vi "Method_Const.vi"(4 "Value":cxt, 5 "Input A":T1) -> (1 "Result":T1)   [LabVIEW 2021, in "Multiply_CPLX_EXT.lvclass"]
uses:
  Multiply_CPLX_EXT.lvclass
  Abs_Type.ctl
  Abs_Types/Complex Extended Float/Abs_Complex Extended Float.lvclass
  C:/Program Files (x86)/National Instruments/LabVIEW 2021/vi.lib/TSA/Abstract Data Classes/Abs_Types/Numeric/Abs_Numeric.lvclass
  C:/TSA/LV_Abstract/Source/Functions/Support/Function/Two Terminal/Cmplx EXT/AbsFunc_Two Term_Complex EXT.lvclass
  C:/Program Files (x86)/National Instruments/LabVIEW 2021/vi.lib/TSA/Abstract Data Classes/Abs_Types/Complex Extended Float/Abs_Complex Extended Float.lvclass
  Support/Function/Two Terminal/Cmplx EXT/AbsFunc_Two Term_Complex EXT.lvclass/AbsFunc_Two Term_Complex EXT.ctl
  Support/Function/Two Terminal/Cmplx EXT/Properties/Write Numeric A.vi
  Support/Function/Two Terminal/Cmplx EXT/Properties/Write Numeric B.vi
  Constants/Support/CPLX_EXT/Const_CPLX_EXT.lvclass
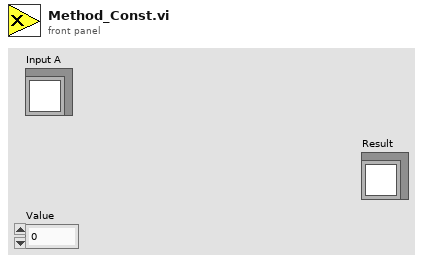
[diagram p1: front panel]
types:
  T1 = typedef "Multiply_CPLX_EXT.lvclass/Abs_Type.ctl" = refnum<class "Abs_Complex Extended Float.lvclass">
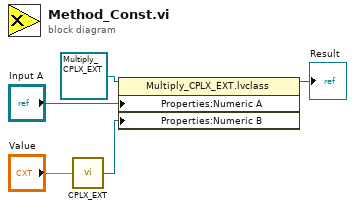
[diagram p0: block diagram]
diagram:
  n1 = call "CPLX_EXT.vi"("Value"="Value") -> ("Constant"=w2:refnum<class "Abs_Complex Extended Float.lvclass">)  [unwired: 4 in]
  n2 = property class="Multiply_CPLX_EXT.lvclass"(reference=refnum<class "Multiply_CPLX_EXT.lvclass"> refnum ("Functions.lvlib:Numeric.lvlib:Multiply.lvclass"), "Properties:Numeric A"="Input A", "Properties:Numeric B"=w2) -> (reference out=→"Result":refnum<class "Multiply_CPLX_EXT.lvclass">)  [unwired: 1 in, 1 out]
